vi "Benchmark SV Receive LV2012 - NI Verified - 100 Byte - PC - 1Var.vi"() -> ()   [LabVIEW 2015]
panel:
  out "Counter":i32
  out "Average Delay (ms)":dbl
  out "Delay (ms)":u32
  out "appended array":i32[][](array[numeric])
  in  "100 byte 2":i32[][](array[numeric])=[[0, 0, 0, 0, 0, 0, 0, 0, 0, 0], [0, 0, 0, 0, 0, 0, 0, 0, 0, 0], [0, 0, 0, 0, 0, 0, 0, 0, 0, 0], [0, 0, 0, 0, 0, 0, 0, 0, 0, 0], [0, 0, 0, 0, 0, 0, 0, 0, 0, 0], [0, 0, 0, 0, 0, 0, 0, 0, 0, 0], [0, 0, 0, 0, 0, 0, 0, 0, 0, 0], [0, 0, 0, 0, 0, 0, 0, 0, 0, 0], [0, 0, 0, 0, 0, 0, 0, 0, 0, 0], [0, 0, 0, 0, 0, 0, 0, 0, 0, 0]]
  out "100 byte":i32[][](array[numeric])
  in  "stop":bool
  # "Overview:  Coding that exemplifies how to benchmark the communication of Shared Variables.\nRequirements: LabVIEW 2012 or compatible\nInstructions:\n1. Run this VI\n2. Watch the amount of time it takes to communicate on the \"Benchmark SV Send  LV2012 - NI Verified.vi\" \n3. Stop both VIs"
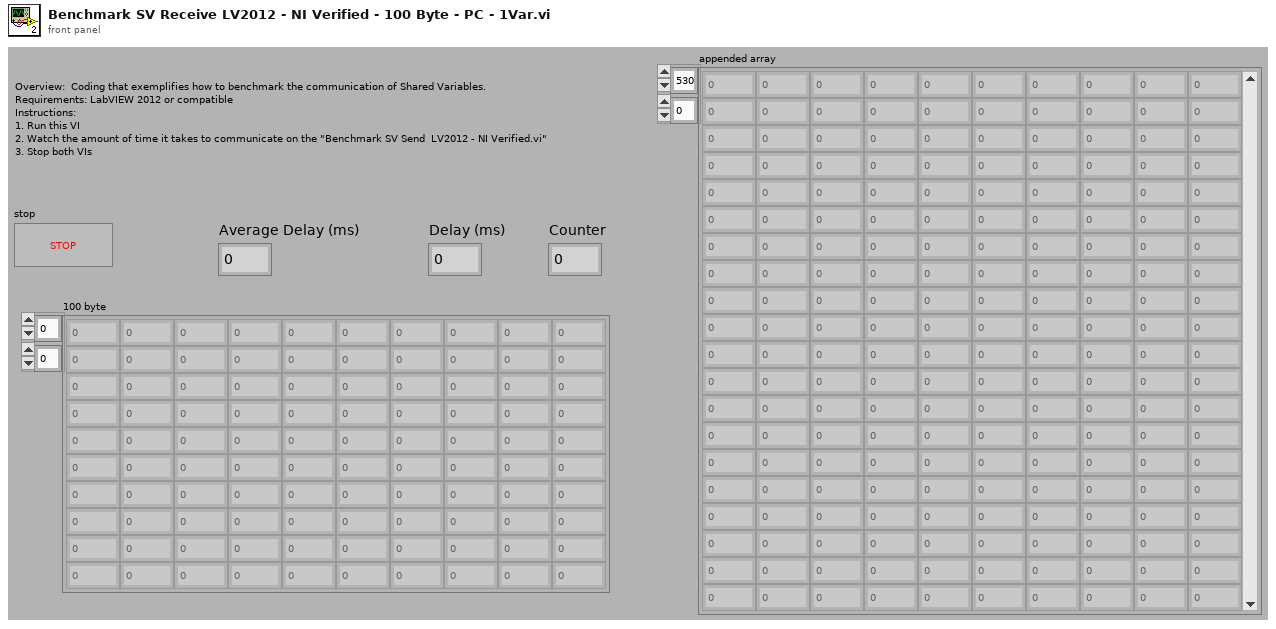
[diagram p1: front panel]
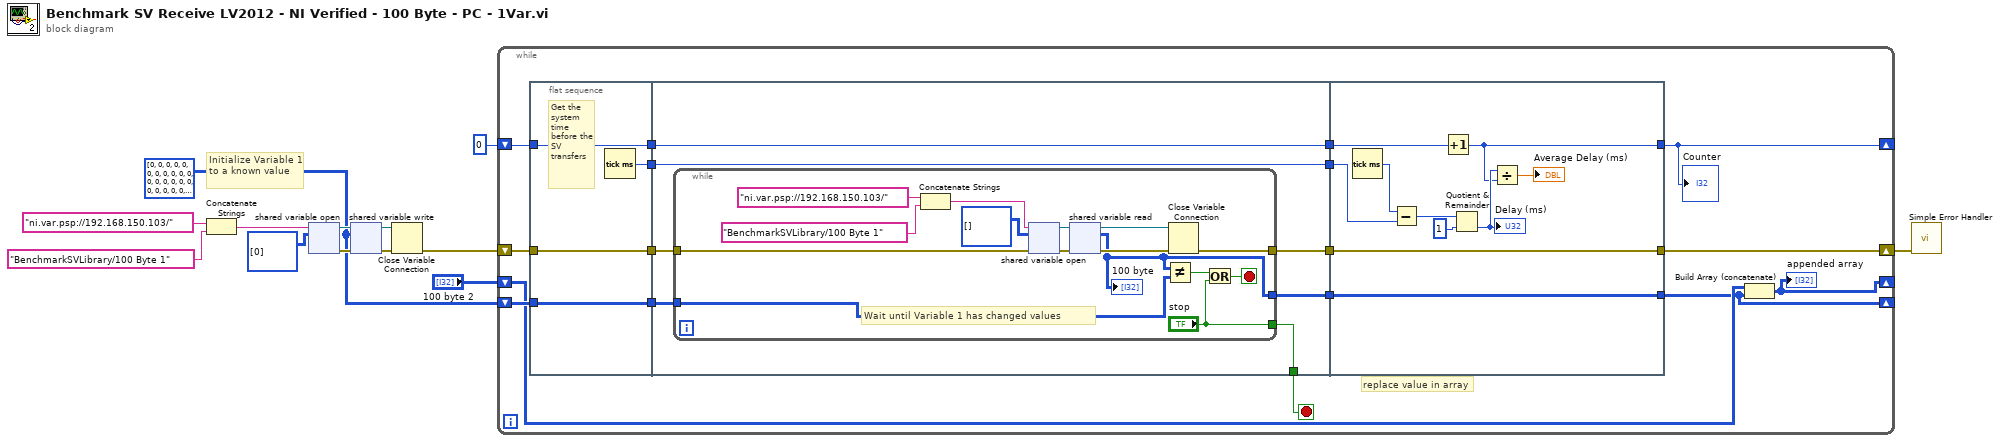
[diagram p0: block diagram]
diagram:
  w2 = i32[][] [[0, 0, 0, 0, 0, 0, 0, 0, 0, 0], [0, 0, 0, 0, 0, 0, 0, 0, 0, 0], [0, 0, 0, 0, 0, 0, 0, 0, 0, 0], [0, 0, 0, 0, 0, 0, 0, 0, 0, 0], [0, 0, 0, 0, 0, 0, 0, 0, 0, 0], [0, 0, 0, 0, 0, 0, 0, 0, 0, 0], [0, 0, 0, 0, 0, 0, 0, 0, 0, 0], [0, 0, 0, 0, 0, 0, 0, 0, 0, 0], [0, 0, 0, 0, 0, 0, 0, 0, 0, 0], [0, 0, 0, 0, 0, 0, 0, 0, 0, 0]] ("appended array")
  # "Initialize Variable 1 to a known value"
  n1 = Concatenate Strings("ni.var.psp://192.168.150.103/" ("string"), "BenchmarkSVLibrary/100 Byte 1") -> (w12:string)
  n2 = shared-variable-open(w12, i32[][] [[0]] ("appended array")) -> (w10:refnum<k21>, w8:errorcluster)  [unwired: 2 in]
  n3 = shared-variable-write(w10, w8, w2) -> (w9:refnum<k21>, w7:errorcluster)
  n4 = Close Variable Connection(8:w7, 11:w9) -> (0:w6:errorcluster)
  n5 = while {
    shift-right: [w29] -> w13
    shift-left: w6 -> [w30]
    shift-right: [w28] -> _
    shift-left: "100 byte 2" -> [w26]
    shift-right: [w25] -> _
    shift-left: w2 -> [w27]
    shift-right: [w14] -> _
    shift-left: 0 -> [w15]
    stop <- w24 stop-if-true
    # "replace value in array"
    n6 = flat-sequence {
      tunnel: w27 -> [w33]
      tunnel: w30 -> [w34]
      tunnel: [w34] -> w23
      tunnel: [w33] -> w22
      tunnel: [w32] -> w18
      tunnel: [w31] -> w16
      tunnel: w15 -> [w31]
      tunnel: [w37] -> w24
      tunnel: w23 -> [w41]
      tunnel: w22 -> [w39]
      tunnel: [w40] -> w21
      tunnel: [w38] -> w20
      tunnel: [w36] -> w19
      tunnel: w18 -> [w36]
      tunnel: [w35] -> w17
      tunnel: w16 -> [w35]
      tunnel: [w65] -> w25
      tunnel: [w66] -> w29
      tunnel: w21 -> [w66]
      tunnel: w20 -> [w65]
      tunnel: w19 -> [w59]
      tunnel: w17 -> [w58]
      tunnel: [w57] -> w14
      frame #0 {
        # "Get the system time before the SV transfers"
        n7 = Tick Count (ms)() -> (millisecond timer value=w32:u32)
      }
      frame #1 {
        n8 = while {
          tunnel: [w43] -> w38
          tunnel: ["stop"] -> w37
          tunnel: [w48] -> w40
          tunnel: w41 -> [w47]
          tunnel: w39 -> [w42]
          stop <- w54 stop-if-true
          # "Wait until Variable 1 has changed values"
          n9 = Concatenate Strings("ni.var.psp://192.168.150.103/" ("string"), "BenchmarkSVLibrary/100 Byte 1") -> (w44:string)
          n10 = shared-variable-open(w44, w47, i32[][] [] ("appended array")) -> (w52:refnum<k21>, w51:errorcluster)  [unwired: 1 in]
          n11 = shared-variable-read(w52, w51) -> (w50:refnum<k21>, w49:errorcluster, w43:i32[][])  [unwired: 1 out]
          "100 byte" <- w43
          n12 = Not Equal?(x=w43, y=w42) -> (x != y?=w56:bool)
          n13 = Close Variable Connection(8:w49, 11:w50) -> (0:w48:errorcluster)
          n14 = Or(x=w56, y="stop") -> (x .or. y?=w54:bool)
        }
      }
      frame #2 {
        n15 = Tick Count (ms)() -> (millisecond timer value=w60:u32)
        n16 = Subtract(x=w60, y=w59) -> (x-y=w62:u32)
        n17 = Increment(x=w58) -> (x+1=w57:i32)
        n18 = Quotient & Remainder(x=w62, y=u32 1) -> (floor(x/y)=w64:u32)  [unwired: 1 out]
        "Delay (ms)" <- w64
        n19 = Divide(x=w64, y=w57) -> (x/y=→"Average Delay (ms)":dbl)
      }
    }
    n20 = Build Array (concatenate)(w26, w25) -> (w28:i32[][])
    "appended array" <- w28
    "Counter" <- w14
  }
  n21 = call <vilib>:"Simple Error Handler.vi"("error in (no error)"=w13) -> ()  [unwired: 4 in, 5 out]
